vi "VI.vi"() -> ()   [LabVIEW 2021]
uses:
  Enum.ctl
  <vilib>/Instr/_visa.llb/VISA Configure Serial Port (Instr).vi
panel:
  out "PH10":cluster{"Output Value":dbl, dbl, dbl}(graph)
  out "p":cluster{"Output Value":dbl, dbl, dbl}(graph)
  out "RH":cluster{"Output Value":dbl, dbl, dbl}(graph)
  out "T":cluster{"Output Value":dbl, dbl, dbl}(graph)
  out "Iteracje Pomiarowe":i32
  out "Zapylenie Srednie Godz [ug/m3]":dbl
  out "Cisnienie Srednie Godz [hPa]":dbl
  out "Wilgotnosc Srednia Godz [%]":dbl
  out "Temperatura Srednia Godz [oC]":dbl
  out "Zapylenie Srednie Min [ug/m3]":dbl
  out "Cisnienie Srednie Min [hPa]":dbl
  out "Wilgotnosc Srednia Min [%]":dbl
  out "Temperatura Srednia Min [oC]":dbl
  out "PH10Array":dbl[](array[numeric])
  out "pArray":dbl[](array[numeric])
  out "RHArray":dbl[](array[numeric])
  out "TArray":dbl[](array[numeric])
  out "Zapylenie [ug/m3]":dbl
  in  "Potwierdz Haslo":bool
  in  "Haslo":string
  out "Cisnienie [hPa]":dbl
  out "Wilgotnosc [%]":dbl
  out "Temperatura [oC]":dbl
  out "Iteracje Programu":i32
  in  "Stop":bool
  in  "Arduino Port":refnum<visa-resource-name>
  # "Stacja Pogodowa"
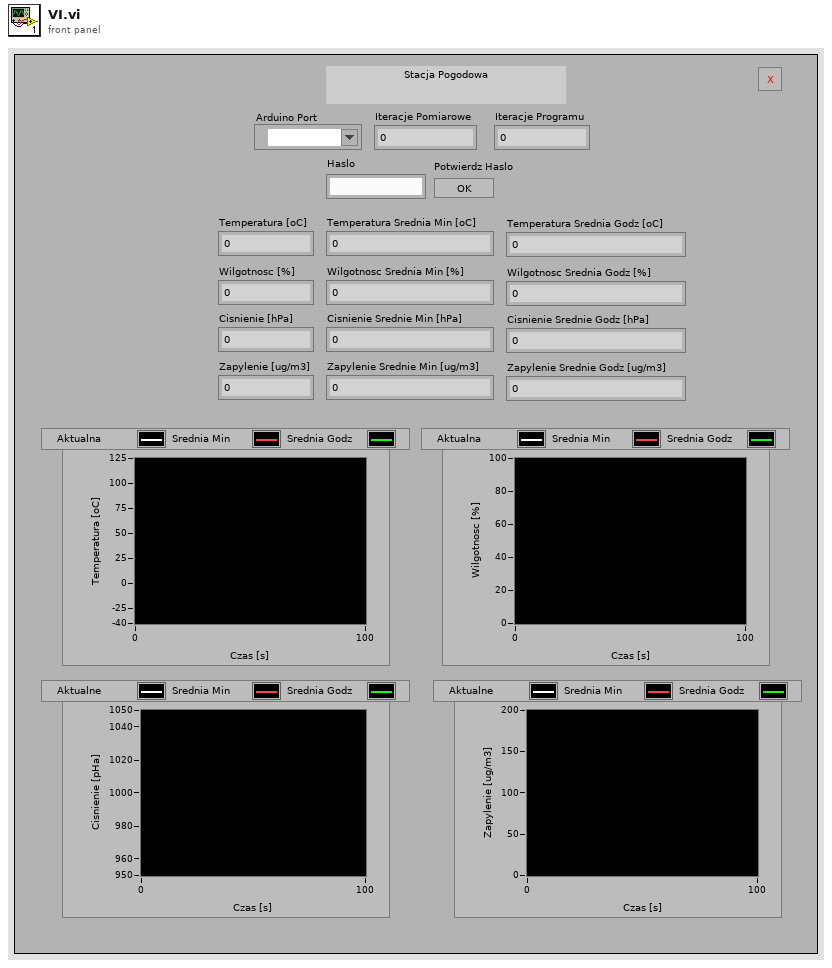
[diagram p1: front panel]
types:
  T1 = typedef "Enum.ctl" = enum16{"Init", "Password", "Measurement", "End"}
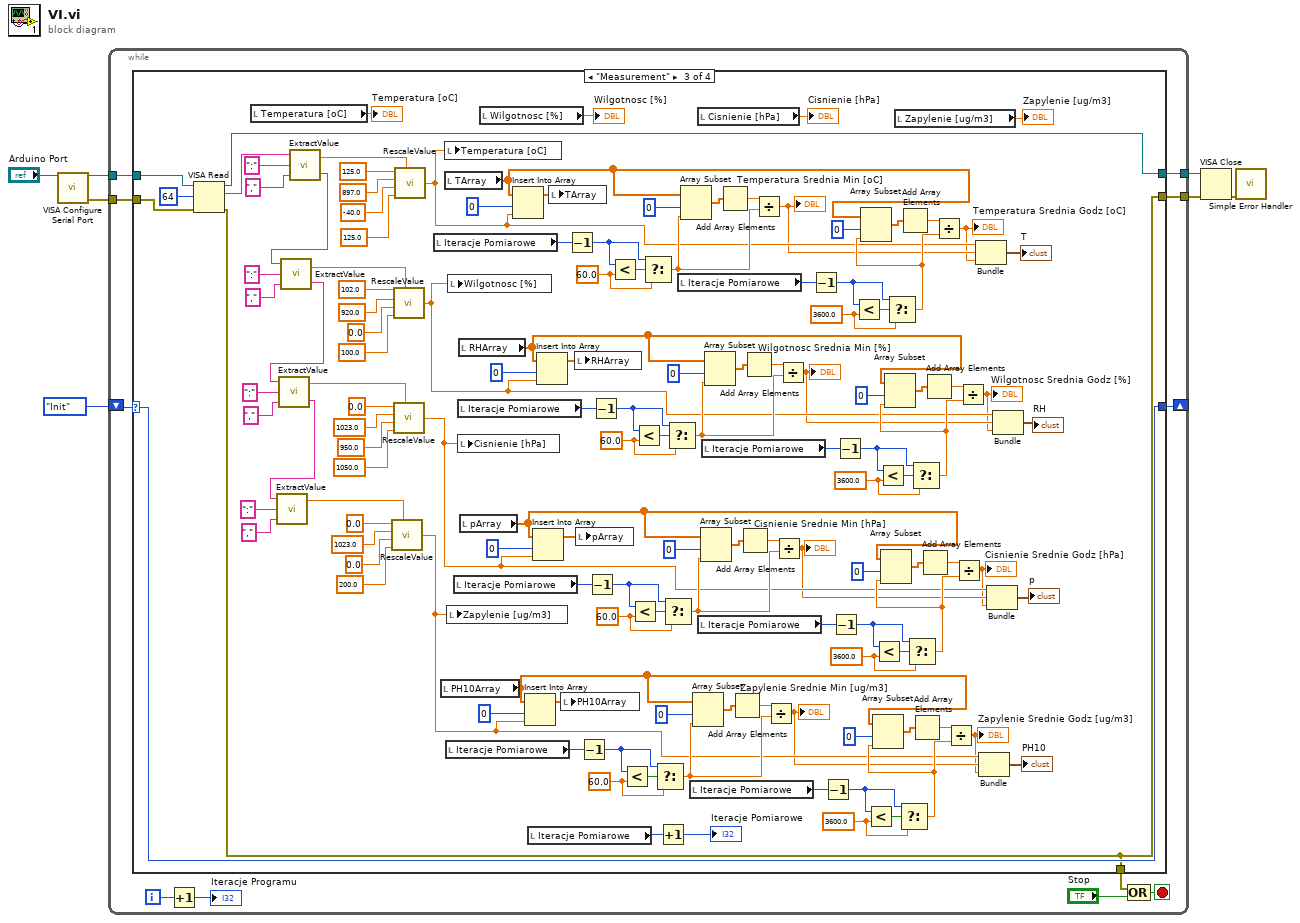
[diagram p0: block diagram]
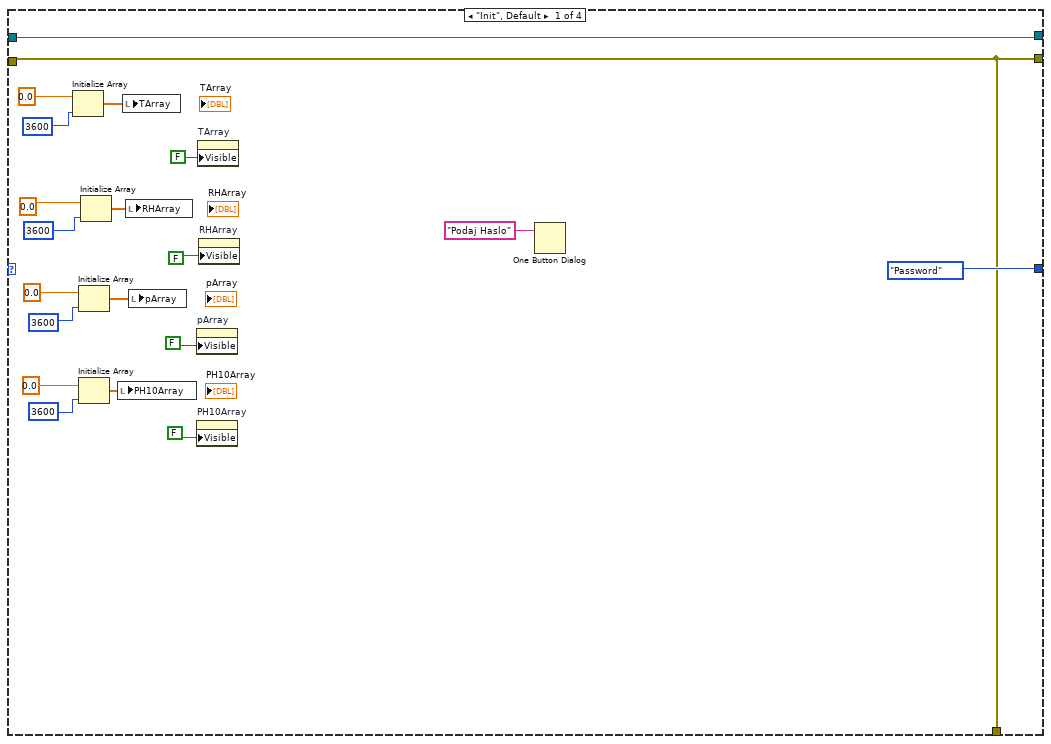
[diagram p2: hidden frame]
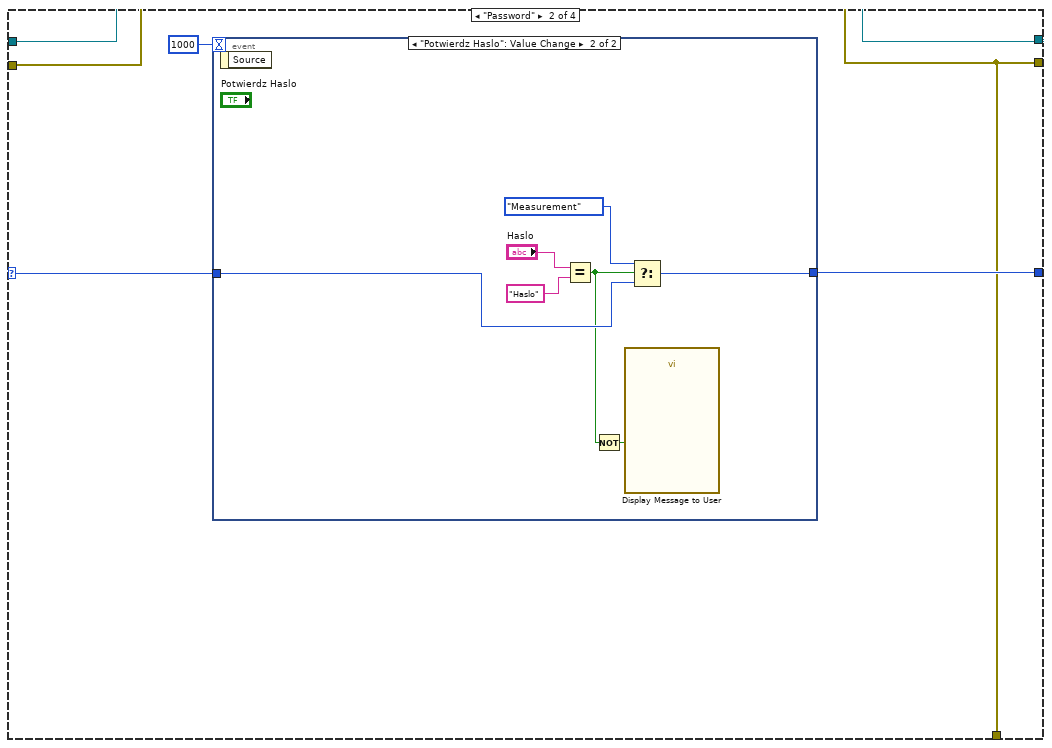
[diagram p3: hidden frame]
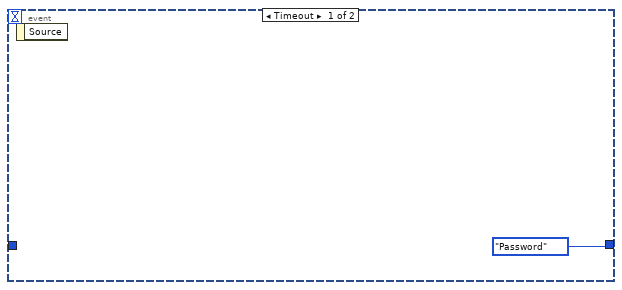
[diagram p4: hidden frame]
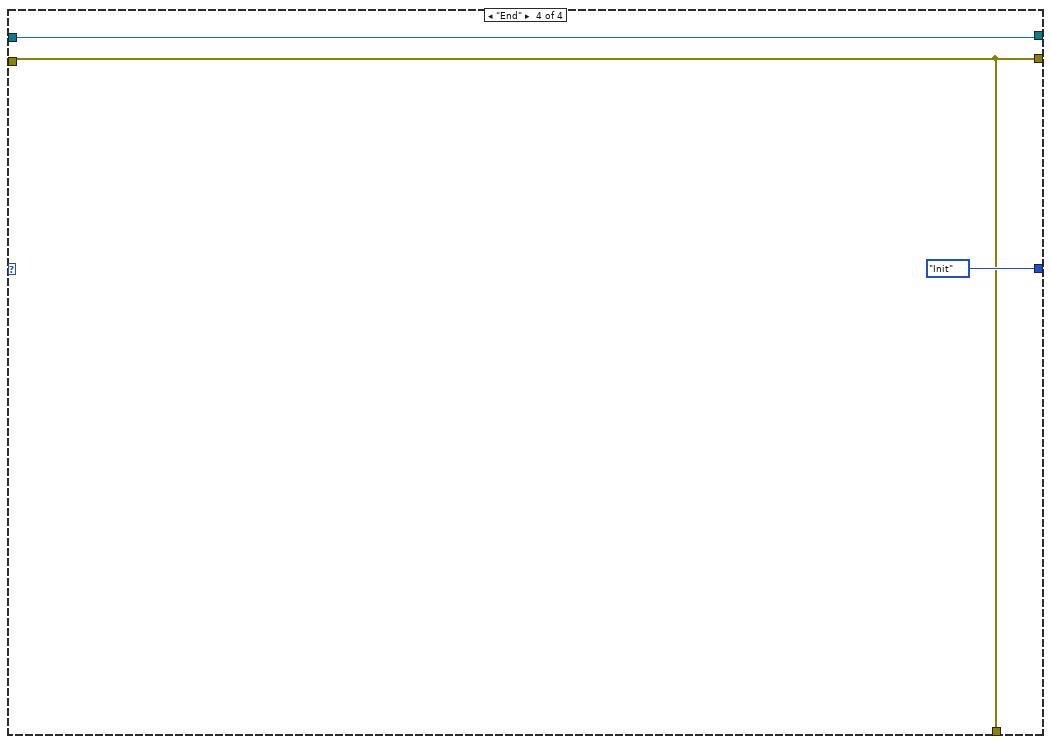
[diagram p5: hidden frame]
diagram:
  n1 = call-poly "VISA Configure Serial Port"("VISA resource name"="Arduino Port") -> ("VISA resource name out"=w7:refnum<visa-resource-name>, "error out"=w6:errorcluster)  [unwired: 13 in]
  n2 = while {
    tunnel: w7 -> [w13]
    tunnel: w6 -> [w11]
    shift-right: [w14] -> _
    shift-left: Enum."Init" ("Enum") -> [w15]
    tunnel: [w12] -> w2
    tunnel: [w10] -> w1
    i -> [w18]
    stop <- w17 stop-if-true
    n3 = case shown="\"Measurement\"" w15 {
      selector: w15 -> [_ w42 w162 _]
      tunnel: [Enum."Password" ("Enum") w41 w162 Enum."Init" ("Enum")] -> w14
      tunnel: w13 -> [w36 w40 w161 w189]
      tunnel: [w36 w40 w68 w189] -> w12
      tunnel: w11 -> [w35 w39 w160 w188]
      tunnel: [w35 w39 w159 w188] -> w10
      tunnel: [w35 w39 w159 w188] -> w9
      frame "Init", Default {
        n4 = Initialize Array(0.0 ("element"), 3600 ("dimension size")) -> (w32:dbl[])
        n5 = Initialize Array(0.0 ("element"), 3600 ("dimension size")) -> (w24:dbl[])
        n6 = Initialize Array(0.0 ("element"), 3600 ("dimension size")) -> (w20:dbl[])
        n7 = Initialize Array(0.0 ("element"), 3600 ("dimension size")) -> (w28:dbl[])
        n8 = local write "PH10Array"(w20) -> ()
        n9 = local write "TArray"(w32) -> ()
        n10 = local write "RHArray"(w28) -> ()
        n11 = local write "pArray"(w24) -> ()
        n12 = property on="pArray" class="Arr (strict)"("Visible"=FALSE) -> ()  [unwired: 2 in, 2 out]
        n13 = property on="PH10Array" class="Arr (strict)"("Visible"=FALSE) -> ()  [unwired: 2 in, 2 out]
        n14 = property on="TArray" class="Arr (strict)"("Visible"=FALSE) -> ()  [unwired: 2 in, 2 out]
        n15 = property on="RHArray" class="Arr (strict)"("Visible"=FALSE) -> ()  [unwired: 2 in, 2 out]
        n16 = One Button Dialog(message="Podaj Haslo") -> ()  [unwired: 1 in, 1 out]
      }
      frame "Password" {
        n17 = event shown="[1] \"Potwierdz Haslo\": Value Change" {
          selector: _ -> [_ _]
          dyn-events: _ -> [_ _]
          timeout: 1000 -> [_ _]
          tunnel: w42 -> [_ w48]
          tunnel: [Enum."Password" ("Enum") w47] -> w41
          event Timeout {
            n18 = event-data() -> ()  [unwired: 1 in, 1 out]
          }
          event "Potwierdz Haslo": Value Change {
            n19 = event-data() -> ()  [unwired: 1 in, 1 out]
            n20 = Equal?(x="Haslo", y="Haslo") -> (x = y?=w46:bool)
            n21 = Not(x=w46) -> (.not. x?=w45:bool)
            n22 = call "Display Message to User"("Enable"=w45) -> ()  [unwired: 9 in, 2 out]
            n23 = Select(t=Enum."Measurement" ("Enum"), s=w46, f=w48) -> (s? t:f=w47:T1)
          }
        }
      }
      frame "Measurement" {
        w76 = 3600.0 ("y")
        w83 = 60.0 ("y")
        w94 = 3600.0 ("y")
        w101 = 60.0 ("y")
        w112 = 3600.0 ("y")
        w119 = 60.0 ("y")
        w131 = 3600.0 ("y")
        w138 = 60.0 ("y")
        n24 = VISA Read(VISA resource name=w161, byte count=u32 64, error in (no error)=w160) -> (VISA resource name out=w68:refnum<visa-resource-name>, read buffer=w184:string, error out=w159:errorcluster)  [unwired: 1 out]
        n25 = local read "Temperatura [oC]"() -> (→"Temperatura [oC]":dbl)
        n26 = call "ExtractValue.vi"("Filter 2"=",", "Filter 1"=":", "Input String"=w184) -> ("Output String"=w187:string, "Output Number"=w186:dbl)
        n27 = call "ExtractValue.vi"("Filter 2"=",", "Filter 1"=":", "Input String"=w187) -> ("Output String"=w183:string, "Output Number"=w185:dbl)
        n28 = call "ExtractValue.vi"("Filter 2"=",", "Filter 1"=":", "Input String"=w183) -> ("Output String"=w148:string, "Output Number"=w182:dbl)
        n29 = call "ExtractValue.vi"("Filter 2"=",", "Filter 1"=":", "Input String"=w148) -> ("Output Number"=w149:dbl)  [unwired: 1 out]
        n30 = call "RescaleValue.vi"("Old Scale Min"=0.0, "Old Scale Max"=1023.0, "New Scale Min"=0.0, "New Scale Max"=200.0, "Input Value"=w149) -> ("Output Value"=w55:dbl)
        n31 = call "RescaleValue.vi"("Old Scale Min"=102.0, "Old Scale Max"=920.0, "New Scale Min"=0.0, "New Scale Max"=100.0, "Input Value"=w185) -> ("Output Value"=w63:dbl)
        n32 = call "RescaleValue.vi"("Old Scale Min"=0.0, "Old Scale Max"=1023.0, "New Scale Min"=950.0, "New Scale Max"=1050.0, "Input Value"=w182) -> ("Output Value"=w59:dbl)
        n33 = call "RescaleValue.vi"("Old Scale Min"=125.0, "Old Scale Max"=897.0, "New Scale Min"=-40.0, "New Scale Max"=125.0, "Input Value"=w186) -> ("Output Value"=w67:dbl)
        n34 = local read "Iteracje Pomiarowe"() -> (w141:i32)
        n35 = local read "PH10Array"() -> (w72:dbl[])
        n36 = local write "Temperatura [oC]"(w67) -> ()
        n37 = local read "TArray"() -> (w127:dbl[])
        n38 = local read "Iteracje Pomiarowe"() -> (w86:i32)
        n39 = local write "Zapylenie [ug/m3]"(w55) -> ()
        n40 = local write "Wilgotnosc [%]"(w63) -> ()
        n41 = local read "Iteracje Pomiarowe"() -> (w104:i32)
        n42 = local read "Iteracje Pomiarowe"() -> (w122:i32)
        n43 = local write "Cisnienie [hPa]"(w59) -> ()
        n44 = local read "RHArray"() -> (w108:dbl[])
        n45 = local read "pArray"() -> (w90:dbl[])
        n46 = local read "Wilgotnosc [%]"() -> (→"Wilgotnosc [%]":dbl)
        n47 = Insert Into Array(array=w127, index=0, new element=w67) -> (w146:dbl[])
        n48 = Insert Into Array(array=w72, index=0, new element=w55) -> (w89:dbl[])
        n49 = local read "Iteracje Pomiarowe"() -> (w143:i32)
        n50 = Insert Into Array(array=w90, index=0, new element=w59) -> (w107:dbl[])
        n51 = Insert Into Array(array=w108, index=0, new element=w63) -> (w125:dbl[])
        n52 = local write "TArray"(w146) -> ()
        n53 = local write "PH10Array"(w89) -> ()
        n54 = Decrement(x=w141) -> (x-1=w139:i32)
        n55 = local write "RHArray"(w125) -> ()
        n56 = local write "pArray"(w107) -> ()
        n57 = Decrement(x=w86) -> (x-1=w84:i32)
        n58 = Decrement(x=w104) -> (x-1=w102:i32)
        n59 = Decrement(x=w122) -> (x-1=w120:i32)
        n60 = Less?(x=w139, y=w138) -> (x < y?=w140:bool)
        n61 = Less?(x=w84, y=w83) -> (x < y?=w85:bool)
        n62 = Less?(x=w102, y=w101) -> (x < y?=w103:bool)
        n63 = Less?(x=w120, y=w119) -> (x < y?=w121:bool)
        n64 = Select(t=w139, s=w140, f=w138) -> (s? t:f=w136:dbl)
        n65 = Select(t=w84, s=w85, f=w83) -> (s? t:f=w81:dbl)
        n66 = Increment(x=w143) -> (x+1=→"Iteracje Pomiarowe":i32)
        n67 = Select(t=w102, s=w103, f=w101) -> (s? t:f=w99:dbl)
        n68 = Select(t=w120, s=w121, f=w119) -> (s? t:f=w117:dbl)
        n69 = local read "Iteracje Pomiarowe"() -> (w134:i32)
        n70 = Array Subset(array=w127, index=0, length=w136) -> (w135:dbl[])
        n71 = local read "Iteracje Pomiarowe"() -> (w79:i32)
        n72 = Array Subset(array=w72, index=0, length=w81) -> (w80:dbl[])
        n73 = local read "Cisnienie [hPa]"() -> (→"Cisnienie [hPa]":dbl)
        n74 = local read "Iteracje Pomiarowe"() -> (w97:i32)
        n75 = Array Subset(array=w90, index=0, length=w99) -> (w98:dbl[])
        n76 = local read "Iteracje Pomiarowe"() -> (w115:i32)
        n77 = Array Subset(array=w108, index=0, length=w117) -> (w116:dbl[])
        n78 = Add Array Elements(numeric array=w135) -> (sum=w142:dbl)
        n79 = Add Array Elements(numeric array=w80) -> (sum=w87:dbl)
        n80 = Add Array Elements(numeric array=w98) -> (sum=w105:dbl)
        n81 = Add Array Elements(numeric array=w116) -> (sum=w123:dbl)
        n82 = Divide(x=w142, y=w136) -> (x/y=w66:dbl)
        "Temperatura Srednia Min [oC]" <- w66
        n83 = Divide(x=w87, y=w81) -> (x/y=w54:dbl)
        "Zapylenie Srednie Min [ug/m3]" <- w54
        n84 = Divide(x=w105, y=w99) -> (x/y=w58:dbl)
        "Cisnienie Srednie Min [hPa]" <- w58
        n85 = Divide(x=w123, y=w117) -> (x/y=w62:dbl)
        "Wilgotnosc Srednia Min [%]" <- w62
        n86 = Decrement(x=w134) -> (x-1=w132:i32)
        n87 = Decrement(x=w79) -> (x-1=w77:i32)
        n88 = Decrement(x=w97) -> (x-1=w95:i32)
        n89 = Decrement(x=w115) -> (x-1=w113:i32)
        n90 = Less?(x=w132, y=w131) -> (x < y?=w133:bool)
        n91 = Less?(x=w77, y=w76) -> (x < y?=w78:bool)
        n92 = Less?(x=w95, y=w94) -> (x < y?=w96:bool)
        n93 = Less?(x=w113, y=w112) -> (x < y?=w114:bool)
        n94 = Select(t=w132, s=w133, f=w131) -> (s? t:f=w126:dbl)
        n95 = Array Subset(array=w127, index=0, length=w126) -> (w128:dbl[])
        n96 = local read "Zapylenie [ug/m3]"() -> (→"Zapylenie [ug/m3]":dbl)
        n97 = Select(t=w77, s=w78, f=w76) -> (s? t:f=w73:dbl)
        n98 = Array Subset(array=w72, index=0, length=w73) -> (w69:dbl[])
        n99 = Add Array Elements(numeric array=w128) -> (sum=w130:dbl)
        n100 = Select(t=w95, s=w96, f=w94) -> (s? t:f=w91:dbl)
        n101 = Array Subset(array=w90, index=0, length=w91) -> (w71:dbl[])
        n102 = Select(t=w113, s=w114, f=w112) -> (s? t:f=w109:dbl)
        n103 = Array Subset(array=w108, index=0, length=w109) -> (w70:dbl[])
        n104 = Add Array Elements(numeric array=w69) -> (sum=w75:dbl)
        n105 = Add Array Elements(numeric array=w71) -> (sum=w93:dbl)
        n106 = Add Array Elements(numeric array=w70) -> (sum=w111:dbl)
        n107 = Divide(x=w130, y=w126) -> (x/y=w65:dbl)
        "Temperatura Srednia Godz [oC]" <- w65
        n108 = Divide(x=w75, y=w73) -> (x/y=w53:dbl)
        "Zapylenie Srednie Godz [ug/m3]" <- w53
        n109 = Divide(x=w93, y=w91) -> (x/y=w57:dbl)
        "Cisnienie Srednie Godz [hPa]" <- w57
        n110 = Divide(x=w111, y=w109) -> (x/y=w61:dbl)
        "Wilgotnosc Srednia Godz [%]" <- w61
        n111 = Bundle("Output Value"=w67, w66, w65) -> (→"T":cluster{"Output Value":dbl, dbl, dbl})  [unwired: 1 in]
        n112 = Bundle("Output Value"=w55, w54, w53) -> (→"PH10":cluster{"Output Value":dbl, dbl, dbl})  [unwired: 1 in]
        n113 = Bundle("Output Value"=w59, w58, w57) -> (→"p":cluster{"Output Value":dbl, dbl, dbl})  [unwired: 1 in]
        n114 = Bundle("Output Value"=w63, w62, w61) -> (→"RH":cluster{"Output Value":dbl, dbl, dbl})  [unwired: 1 in]
      }
      frame "End" {
      }
    }
    n115 = Increment(x=w18) -> (x+1=→"Iteracje Programu":i32)
    n116 = Compound Arithmetic op=OR(w9, "Stop") -> (w17:bool)
  }
  n117 = VISA Close(VISA resource name=w2, error in (no error)=w1) -> (error out=w5:errorcluster)
  n118 = call <vilib>:"Simple Error Handler.vi"("error in (no error)"=w5) -> ()  [unwired: 4 in, 5 out]
